vi "Initialize Values.vi"(8 "error in (no error)":errorcluster, 11 "Relev in":refnum<class "Relev.lvclass">) -> (0 "error out":errorcluster, 3 "Relev out":refnum<class "Relev.lvclass">)   [LabVIEW 2014, in "SeqLoop.lvlib" / "STEP Classes.lvlib" / "Relev.lvclass"]
uses:
  Relev.lvclass
  Relev.lvclass/Relev.ctl
  STEP/STEP.lvclass
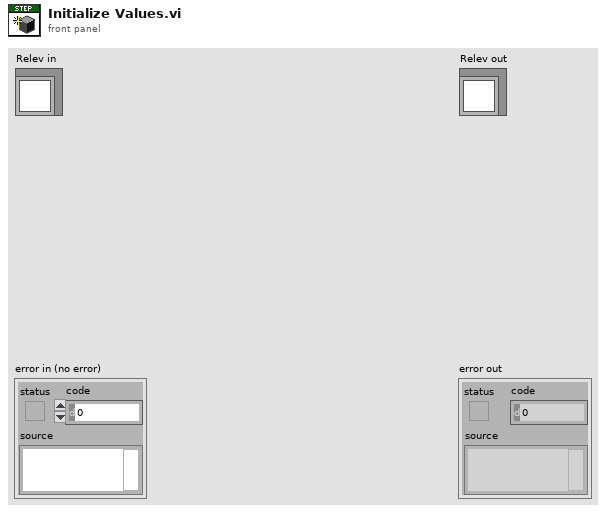
[diagram p1: front panel]
types:
  T1 = cluster{"HWSync 1":bool, "HWSync 2":bool, "HWSync 3":bool, "HWSync 4":bool, "HWSync 5":bool}
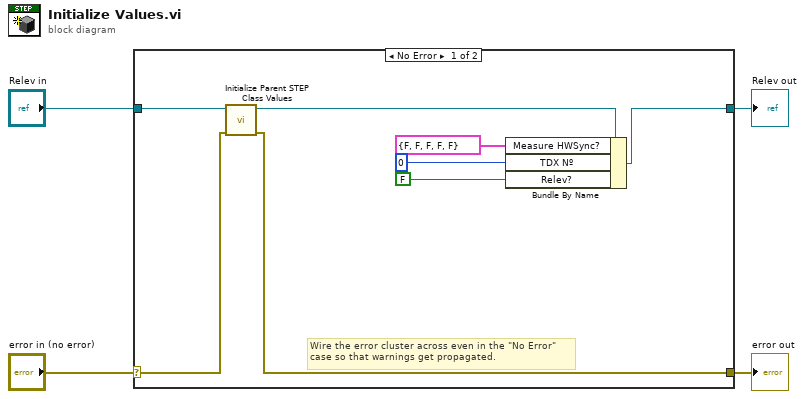
[diagram p0: block diagram]
diagram:
  n1 = case shown="No Error" "error in (no error)" {
    selector: "error in (no error)" -> [w11 w14]
    tunnel: [w10 w14] -> w3
    tunnel: [w8 w13] -> w1
    tunnel: "Relev in" -> [w12 w13]
    frame No Error {
      # "Wire the error cluster across even in the \"No Error\"\ncase so that warnings get propagated."
      n2 = call "Initialize Parent STEP Class Values.vi"("error in (no error)"=w11, "STEP in"=w12) -> ("error out"=w10:errorcluster, "STEP out"=w9:refnum<class "Relev.lvclass">)  [unwired: 8 in]
      n3 = Bundle By Name(cluster=w9, "Measure HWSync?"=T1 {"HWSync 1"=FALSE, "HWSync 2"=FALSE, "HWSync 3"=FALSE, "HWSync 4"=FALSE, "HWSync 5"=FALSE}, "TDX Nº"=0, "Relev?"=FALSE) -> (w8:refnum<class "Relev.lvclass">)
    }
    frame Error {
    }
  }
  "error out" <- w3
  "Relev out" <- w1
